vi "Normalise Input.vi"(11 "Value":i16) -> (3 "Value (Normalised)":sgl)   [LabVIEW 2019, in "SDL2 Utility.lvlib" / "PS4 Controller.lvclass"]
uses:
  PS4 Controller.lvclass
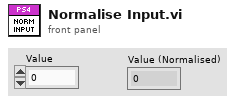
[diagram p1: front panel]
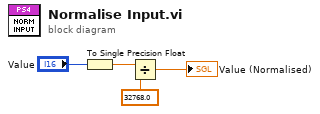
[diagram p0: block diagram]
diagram:
  n1 = To Single Precision Float(number="Value") -> (single precision float=w3:sgl)
  n2 = Divide(x=w3, y=sgl 32768.0) -> (x/y=→"Value (Normalised)":sgl)
